vi "Sort Complex Number Multiplicity (Real).vi"(8 "tolerance":dbl=1e-05, 11 "Complex numbers":cdb[](array[numeric]) format="%#.6f") -> (0 "Multiplicity":i32[](array[numeric]), 3 "Sorted unique complex numbers":cdb[](array[numeric]) format="%#.6f")   [LabVIEW 2020, in "NI_AALPro.lvlib"]
uses:
  <vilib>/Analysis/NI_AALPro.lvlib
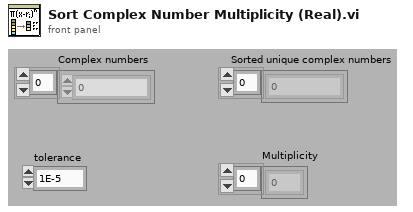
[diagram p1: front panel]
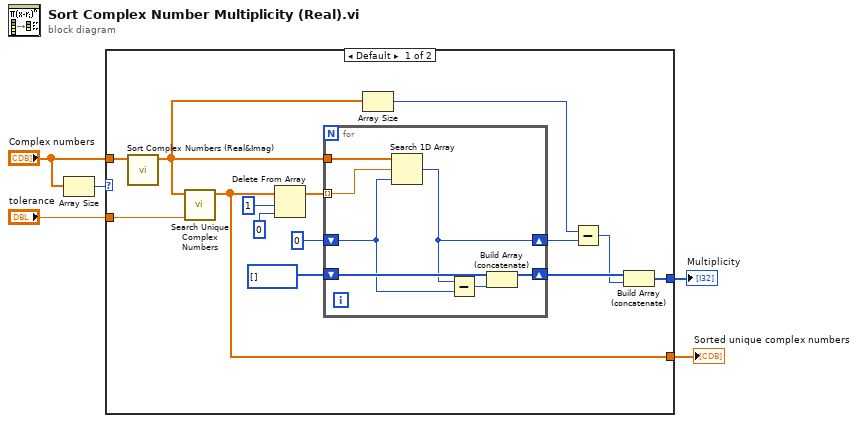
[diagram p0: block diagram]
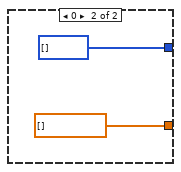
[diagram p2: hidden frame]
diagram:
  n1 = Array Size(array="Complex numbers") -> (size(s)=w2:i32)
  n2 = case shown="Default" w2 {
    tunnel: "Complex numbers" -> [w19 _]
    tunnel: "tolerance" -> [w18 _]
    tunnel: [w15 cdb[] [] ("Unique numbers")] -> w4
    tunnel: [w6 i32[] []] -> w3
    frame Default {
      n3 = call <vilib>:"Sort Complex Numbers (Real&Imag).vi"("Complex Numbers"=w19) -> ("Sorted Complex Numbers"=w11:cdb[])  [unwired: 8 in, 2 out]
      n4 = call <vilib>:"Search Unique Complex Numbers.vi"("tolerance"=w18, "Sorted numbers"=w11) -> ("Unique numbers"=w15:cdb[])  [unwired: 9 in]
      n5 = Delete From Array(array=w15, length=1, index=0) -> (array with subset deleted=w12:cdb[])  [unwired: 1 out]
      n6 = for {
        tunnel: w12 -> [w25] mode=indexing
        tunnel: w11 -> [w26]
        shift-right: [w22] -> w9
        shift-left: 0 -> [w21]
        shift-right: [w23] -> w8
        shift-left: i32[] [] -> [w24]
        n7 = Search 1D Array(1D array=w26, element=w25, start index (0)=w21) -> (index of element=w22:i32)
        n8 = Subtract(x=w22, y=w21) -> (x-y=w20:i32)
        n9 = Build Array (concatenate)(w24, w20) -> (w23:i32[])
      }
      n10 = Array Size(array=w11) -> (size(s)=w10:i32)
      n11 = Subtract(x=w10, y=w9) -> (x-y=w7:i32)
      n12 = Build Array (concatenate)(w8, w7) -> (w6:i32[])
    }
    frame 0 {
    }
  }
  "Sorted unique complex numbers" <- w4
  "Multiplicity" <- w3
